vi "SlewRateLimiter_Close.vi"(11 "out SLEW_RATE_LIMITER":T1 {"NegativeRateLimit" format="%13.5p"; "PrevTime" format="%30.5p"; "PrevValue" format="%13.5p"; "PositiveRateLimit" format="%13.5p"}) -> ()   [LabVIEW 2019, in "Trajectory_Library.lvlib"]
doc: "Releases resources used by a SlewRateLimiter data cluster. \n\n(Since the Timer was removed, this no longer needs to be called. This is now a do nothing function.)\n\n\nInputs:\n - in Slew Rate Limiter -- The Slew Rate Limiter data cluster"
uses:
  Trajectory_Library.lvlib
  TypeDef/SLEW_RATE_LIMITER.ctl
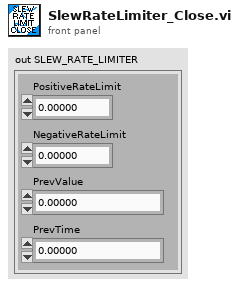
[diagram p1: front panel]
types:
  T1 = typedef "Trajectory_Library.lvlib/SLEW_RATE_LIMITER.ctl" = cluster{"PositiveRateLimit":dbl, "PrevValue":dbl, "PrevTime":dbl, "NegativeRateLimit":dbl}
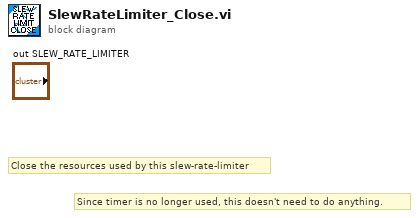
[diagram p0: block diagram]
diagram:
  # "Since timer is no longer used, this doesn't need to do anything."
  # "Close the resources used by this slew-rate-limiter"
